vi "Get Selected Axis.vi"(11 "Axis Array":bool[](array[boolean])) -> (3 "Axis Index":i32)   [LabVIEW 2020, in "Dashboard.lvlib"]
uses:
  Dashboard.lvlib
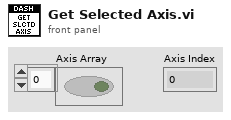
[diagram p1: front panel]
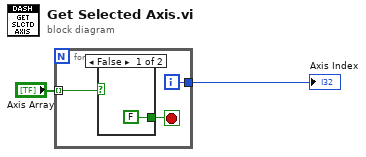
[diagram p0: block diagram]
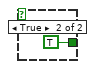
[diagram p2: hidden frame]
diagram:
  n1 = for {
    tunnel: "Axis Array" -> [w5] mode=indexing
    tunnel: [w3] -> w2
    i -> [w3]
    stop <- w4 stop-if-true
    n2 = case shown="False" w5 {
      tunnel: [FALSE TRUE] -> w4
      frame False {
      }
      frame True {
      }
    }
  }
  "Axis Index" <- w2
